vi "Video Processor Create.vi"(4 "Num Threads (-1: CPU count)":i32=-1, 5 "Identifier":string, 6 "Depth History Size (10)":i32=10, 7 "Loop? (T)":bool=TRUE, 8 "error in (no error)":errorcluster, 9 "Open File? (T)":bool=TRUE, 10 "Video Path (\"\")":path, 11 "Video Processor in":refnum<class "Video Processor.lvclass">) -> (0 "error out":errorcluster, 3 "Video Processor out":refnum<class "Video Processor.lvclass">)   [LabVIEW 2018, in "Video Processor.lvclass"]
uses:
  Video Processor.lvclass
  C:/Users/aaron.jencks/Documents/GitHub/emerson_seed_object_detection/LabVIEW/Projects/Paul's Video Viewer/Classes/Video File/Video File.lvclass
  Video Processor.lvclass/Video Processor.ctl
  Video File/Video File.lvclass
  <vilib>/vision/NI_Vision_Development_Module.lvlib
  Standard Averager/Standard Averager.lvclass
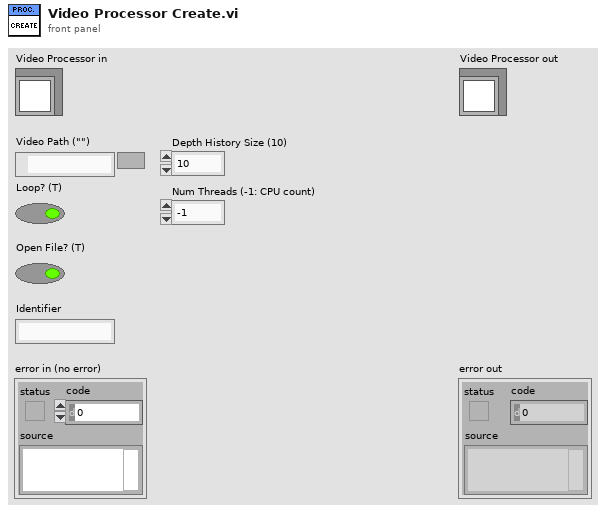
[diagram p1: front panel]
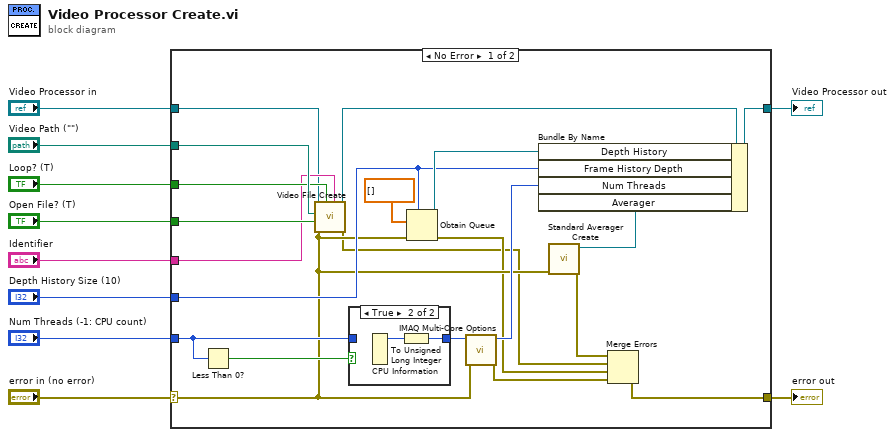
[diagram p0: block diagram]
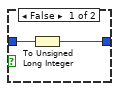
[diagram p2: hidden frame]
diagram:
  n1 = case shown="No Error" "error in (no error)" {
    selector: "error in (no error)" -> [w16 w37]
    tunnel: [w11 w37] -> w9
    tunnel: [w25 w36] -> w7
    tunnel: "Video Processor in" -> [w27 w36]
    tunnel: "Video Path (\"\")" -> [w31 _]
    tunnel: "Loop? (T)" -> [w29 _]
    tunnel: "Open File? (T)" -> [w30 _]
    tunnel: "Identifier" -> [w28 _]
    tunnel: "Depth History Size (10)" -> [w23 _]
    tunnel: "Num Threads (-1: CPU count)" -> [w19 _]
    frame No Error {
      n2 = Less Than 0?(x=w19) -> (x < 0?=w20:bool)
      n3 = call "Video File Create.vi"("Identifier"=w28, "Loop? (T)"=w29, "error in (no error)"=w16, "Open File? (T)"=w30, "Video Path (\"\")"=w31, "Video File in"=w27) -> ("error out"=w13:errorcluster, "Video File out"=w26:refnum<class "Video Processor.lvclass">)  [unwired: 4 in]
      n4 = case shown="True" w20 {
        tunnel: w19 -> [w33 _]
        tunnel: [w32 w34] -> w18
        frame False {
          n5 = To Unsigned Long Integer(number=w33) -> (unsigned 32bit integer=w32:u32)
        }
        frame True {
          n6 = CPU Information() -> (4:w35:i32)  [unwired: 3 out]
          n7 = To Unsigned Long Integer(number=w35) -> (unsigned 32bit integer=w34:u32)
        }
      }
      n8 = Obtain Queue(max queue size (-1, unlimited)=w23, element data type=dbl[] [], error in (no error)=w16) -> (queue out=w24:refnum<queue>, error out=w14:errorcluster)  [unwired: 2 in, 1 out]
      n9 = call "IMAQ Multi-Core Options"("error in (no error)"=w16, "Specified Number of Cores"=w18) -> ("error out"=w15:errorcluster, "Cores Utilized"=w21:u32)  [unwired: 8 in]
      n10 = call "Standard Averager Create.vi"("error in (no error)"=w16) -> ("error out"=w12:errorcluster, "Standard Averager out"=w17:refnum<class "Standard Averager.lvclass">)  [unwired: 9 in]
      n11 = Bundle By Name(cluster=w26, "Depth History"=w24, "Frame History Depth"=w23, "Num Threads"=w21, "Averager"=w17) -> (w25:refnum<class "Video Processor.lvclass">)
      n12 = Merge Errors(w12, w13, w14, w15) -> (w11:errorcluster)
    }
    frame Error {
    }
  }
  "error out" <- w9
  "Video Processor out" <- w7
